vi "Get User and Password Event.vi"(8 "Error In":errorcluster) -> (0 "Error Out":errorcluster, 2 "User Data":string[](array[string]), 3 "do":bool)   [LabVIEW 2020]
doc: "Displays a standard dialog box that prompts users to enter information, such as a user name and password.\n--------------------\n\nThis Express VI is configured as follows:\n\nMessage to Display to the User:Enter User Name and Password\nThe inputs are: \nText Entry Box: User Name\nText Entry Box: Password"
uses:
  support/PCT FGV CMD.ctl
  support/Message Queue/Message Queue.lvlib
panel:
  out "power":bool
  in  "Cancel Button":bool
  in  "OK Button":bool
  in  "User":string(combo)
  in  "Password:":string caption="Password"
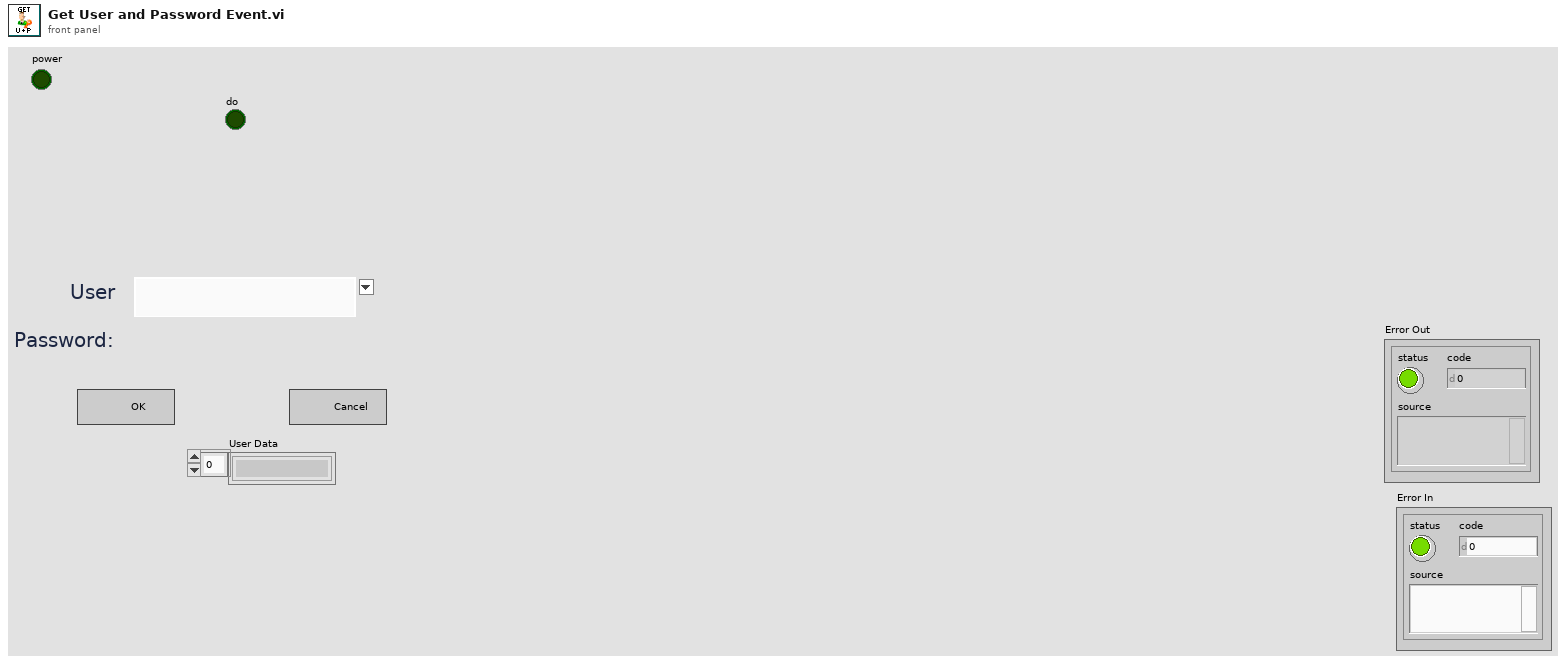
[diagram p1: front panel]
types:
  T1 = typedef "PCT FGV CMD.ctl" = enum16{"INIT", "GET", "SET"}
  T2 = typedef "Message Queue.lvlib/All Message Queues.ctl" = cluster{"UI":refnum<queue>, "Logging":refnum<queue>, "LOG":refnum<queue>, "ALARM":refnum<queue>, "Test":refnum<queue>, "Answer":refnum<queue>, "PLC":refnum<queue>, "DB":refnum<queue>, "Report":refnum<queue>, "OPC":refnum<queue>, "Procedure":refnum<queue>, "PalmSens":refnum<queue>, "SYS 7000 Reader":refnum<queue>, "SWITCH":refnum<queue>, "MOTOR":refnum<queue>, "MOTION":refnum<queue>, "HIDEN":refnum<queue>, "VALVE":refnum<queue>, "MFC":refnum<queue>, "PUMP IN":refnum<queue>, "PUMP OUT":refnum<queue>}
  T3 = cluster{"Type CMD":string, "Mode CMD":string, "Main CMD":string}
  T4 = enum8{"Enabled", "Disabled", "Disabled and Grayed Out"}
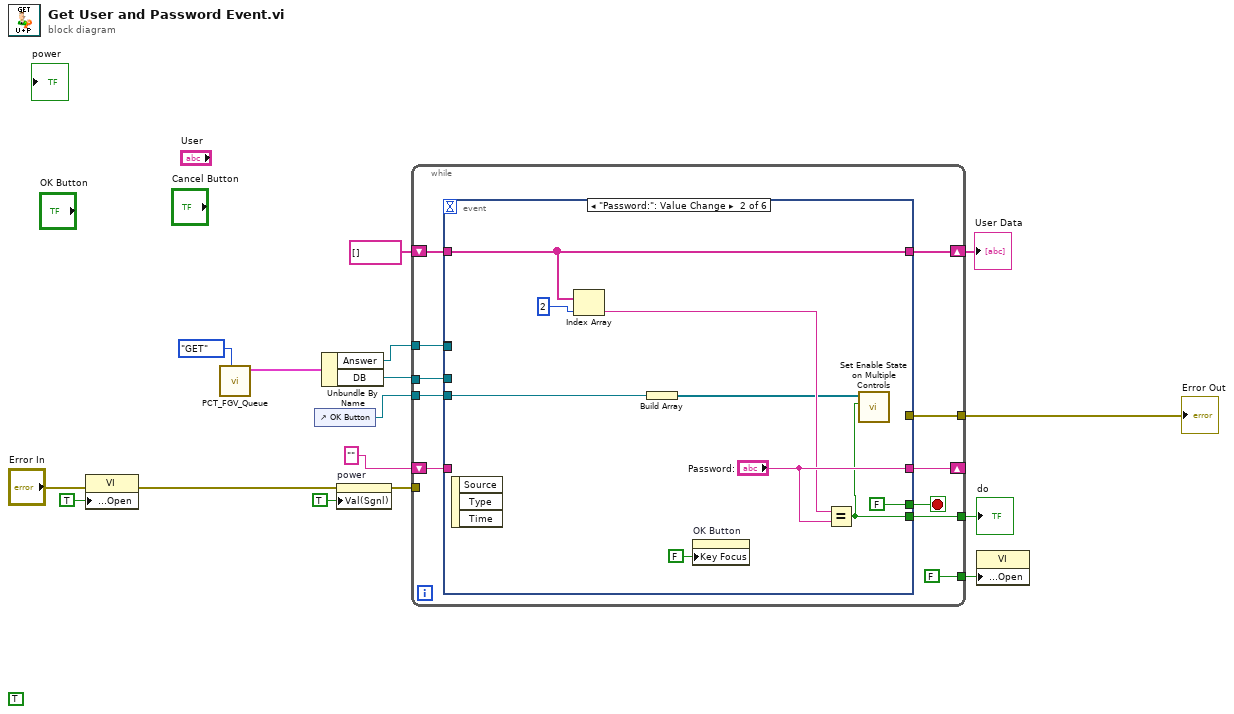
[diagram p0: block diagram]
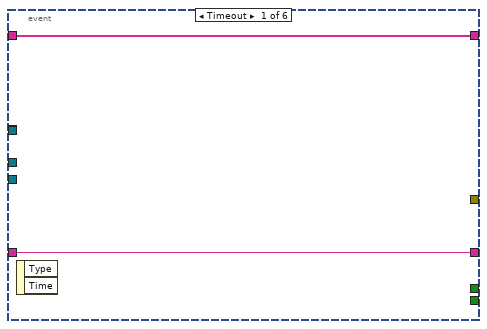
[diagram p2: hidden frame]
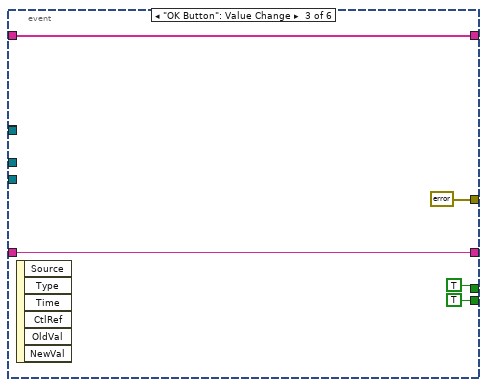
[diagram p3: hidden frame]
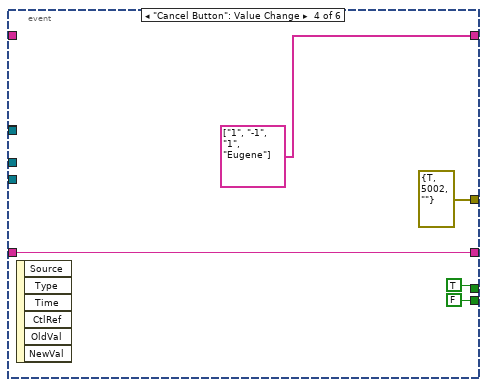
[diagram p4: hidden frame]
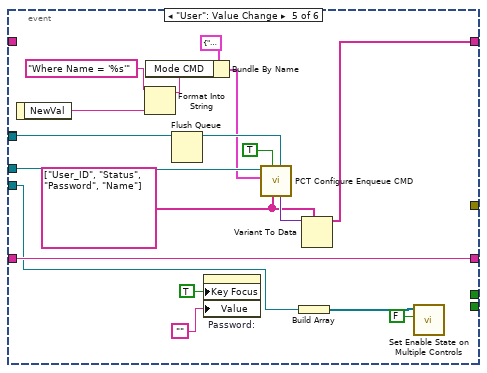
[diagram p5: hidden frame]
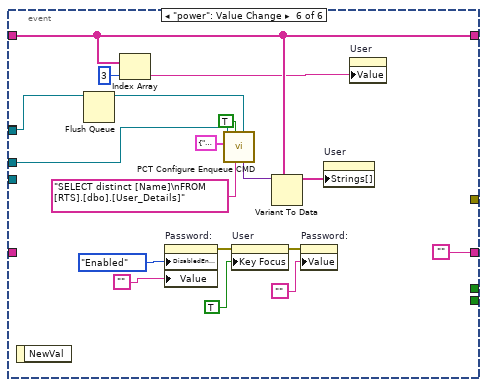
[diagram p6: hidden frame]
diagram:
  (unwired) TRUE ("focus on")
  n1 = property class="VI"(error in="Error In", "Front Panel Window:Open"=TRUE) -> (error out=w14:errorcluster)  [unwired: 1 in, 1 out]
  n2 = call "PCT_FGV_Queue.vi"("CMD"=PCT_FGV_CMD."GET") -> ("Message Queues out"=w9:T2)  [unwired: 9 in, 1 out]
  n3 = control-ref of="OK Button"() -> (w4:refnum<vi>)
  n4 = Unbundle By Name(w9) -> ("Answer"=w8:refnum<queue>, "DB"=w7:refnum<queue>)
  n5 = property on="power" class="Bool (strict)"(error in=w14, "Val(Sgnl)"=TRUE ("Value (Signaling)")) -> (error out=w12:errorcluster)  [unwired: 1 in, 1 out]
  n6 = while {
    shift-right: [w25] -> _
    shift-left: "" ("Password:") -> [w26]
    tunnel: [FALSE ("Front Panel Window:Open")] -> w15
    tunnel: [w23] -> w3
    tunnel: w12 -> [_]
    tunnel: w8 -> [w22]
    shift-right: [w21] -> w5
    shift-left: string[] [] ("User Data in") -> [w20]
    tunnel: w7 -> [w19]
    tunnel: w4 -> [w18]
    tunnel: [w17] -> w1
    stop <- w27 stop-if-true
    n7 = event shown="[1] \"Password:\": Value Change" {
      selector: _ -> [_ _ _ _ _ _]
      dyn-events: _ -> [_ _ _ _ _ _]
      timeout: _ -> [_ _ _ _ _ _]
      tunnel: [_ FALSE TRUE TRUE _ _] -> w27
      tunnel: [w29 "Password:" w44 w49 w62 ""] -> w25
      tunnel: w26 -> [w29 _ w44 w49 w62 _]
      tunnel: [_ w33 TRUE FALSE _ _] -> w23
      tunnel: w22 -> [_ w37 _ _ w60 w81]
      tunnel: [_ w37 _ _ _ _] -> _
      tunnel: [w28 w36 w42 string[] ["1", "-1", "1", "Eugene"] ("User Data") w61 w70] -> w21
      tunnel: w20 -> [w28 w36 w42 _ _ w70]
      tunnel: w19 -> [_ _ _ _ w59 w79]
      tunnel: w18 -> [_ w32 _ _ w58 _]
      tunnel: [_ _ errorcluster {"status"=FALSE, "code"=0, "source"=""} ("Error Out") errorcluster {"status"=TRUE, "code"=5002, "source"=""} ("Error Out") _ _] -> w17
      event Timeout {
        n8 = event-data() -> ()  [unwired: 1 in, 2 out]
      }
      event "Password:": Value Change {
        n9 = event-data() -> ()  [unwired: 1 in, 3 out]
        n10 = Index Array(array=w36, index=2) -> (element=w34:string)
        n11 = Build Array(w32) -> (w31:refnum<vi>[])
        n12 = property on="OK Button" class="Bool"("Key Focus"=FALSE) -> ()  [unwired: 2 in, 2 out]
        n13 = Equal?(x=w34, y="Password:") -> (x = y?=w33:bool)
        n14 = call "Set Enable State on Multiple Controls.vi"("Enable?"=w33, "Controls"=w31) -> ()  [unwired: 9 in, 1 out]
      }
      event "OK Button": Value Change {
        n15 = event-data() -> ()  [unwired: 1 in, 6 out]
      }
      event "Cancel Button": Value Change {
        n16 = event-data() -> ()  [unwired: 1 in, 6 out]
      }
      event "User": Value Change {
        w63 = string[] ["User_ID", "Status", "Password", "Name"]
        n17 = event-data() -> ("NewVal"=w53:string)  [unwired: 1 in]
        n18 = Format Into String(format string="Where Name = '%s'" ("Mode CMD"), w53) -> (resulting string=w54:string)  [unwired: 2 in, 1 out]
        n19 = Bundle By Name(cluster=T3 {"Type CMD"="User_Details", "Mode CMD"="", "Main CMD"="Get Data"} ("CMD"), "Mode CMD"=w54) -> (w56:T3)
        n20 = Flush Queue(queue=w60) -> (queue out=w67:refnum<queue>)  [unwired: 1 in, 2 out]
        n21 = property on="Password:" class="Str"("Key Focus"=TRUE, "Value"="") -> ()  [unwired: 2 in, 2 out]
        n22 = call "PCT Configure Enqueue CMD.vi"("Response Queue"=w67, "Parameter Data"=w63, "Read"=TRUE, "CMD"=w56, "CMD Queue in"=w59) -> ("Message Data"=w64:variant)  [unwired: 4 in, 2 out]
        n23 = Build Array(w58) -> (w57:refnum<vi>[])
        n24 = Variant To Data(type=w63, Variant=w64) -> (data=w61:string[])  [unwired: 1 in, 1 out]
        n25 = call "Set Enable State on Multiple Controls.vi"("Enable?"=FALSE, "Controls"=w57) -> ()  [unwired: 9 in, 1 out]
      }
      event "power": Value Change {
        n26 = event-data() -> ()  [unwired: 1 in, 1 out]
        n27 = Flush Queue(queue=w81) -> (queue out=w80:refnum<queue>)  [unwired: 1 in, 2 out]
        n28 = Index Array(array=w70, index=3) -> (element=w68:string)
        n29 = property on="Password:" class="Str"("DisabledEnum"=T4."Enabled" ("Disabled"), "Value"="") -> (error out=w74:errorcluster)  [unwired: 2 in, 1 out]
        n30 = call "PCT Configure Enqueue CMD.vi"("Response Queue"=w80, "Parameter Data"="SELECT distinct [Name]\nFROM [RTS].[dbo].[User_Details]", "Read"=TRUE, "CMD"=T3 {"Type CMD"="User_Name", "Mode CMD"="Swept SA", "Main CMD"="Get Data"}, "CMD Queue in"=w79) -> ("Message Data"=w83:variant)  [unwired: 4 in, 2 out]
        n31 = property on="User" class="CmbBox"(error in=w74, "Key Focus"=TRUE) -> (error out=w76:errorcluster)  [unwired: 1 in, 1 out]
        n32 = Variant To Data(type=w70, Variant=w83) -> (data=w77:string[])  [unwired: 1 in, 1 out]
        n33 = property on="Password:" class="Str"(error in=w76, "Value"="") -> ()  [unwired: 1 in, 2 out]
        n34 = property on="User" class="CmbBox"("Strings[]"=w77) -> ()  [unwired: 2 in, 2 out]
        n35 = property on="User" class="CmbBox"("Value"=w68) -> ()  [unwired: 2 in, 2 out]
      }
    }
  }
  "Error Out" <- w1
  "do" <- w3
  "User Data" <- w5
  n36 = property class="VI"("Front Panel Window:Open"=w15) -> ()  [unwired: 2 in, 2 out]
